vi "AguaClara Design Tool.vi"() -> ()   [LabVIEW 2015, in "AguaClara Library.lvlib"]
uses:
  AguaClara Library.lvlib
  Project commands.ctl
  language cmd.ctl
  Language.ctl
  User status cmd.ctl
  ADT Commands.ctl
  <vilib>/Utility/config.llb/NI_LVConfig.lvlib
  <vilib>/Utility/config.llb/Write Key (I32).vi
  <vilib>/Utility/config.llb/Read Key (I32).vi
  GUI controls commands.ctl
  <vilib>/Platform/browser.llb/Open URL in Default Browser (string).vi
  Project inputs.ctl
  toolbar icons/help.ctl
  User Information.ctl
  Basic Inputs.ctl
  Country Ring.ctl
panel:
  out "Quit now":bool caption="Terminar"
  in  "MSG Server unavailable":string caption="Disculpe. El servidor de AguaClara no está disponible."
  in  "MSG Design sent postcity":string caption="se ha enviado al servidor de AguaClara para el diseño. Los archivos serán enviados a su correo electrónico."
  in  "MSG Design sent precity":string caption="Su solicitude para la ciudad de"
  out "Design Inputs Label":string caption="Datos basicos"
  out "Project Info label":string caption="Información del proyecto"
  in  "Design Plant":bool caption="Mandar la solicitud"
  in  "Logon":bool caption="Entrar al sistema"
  in  "Log off":bool caption="Cierre la sesión"
  in  "Quit":bool caption="Terminar"
  in  "Project commands":T1 caption="Mandados del proyecto"
  in  "Project List":i32(listbox)=-1 caption="Lista de proyectos"
  in  "Help Button":T2 caption="Botón para ayuda"
  in  "Tab Control":enum32{" ", "  ", "Advanced Controls"}(tab)=enum."Advanced Controls" caption="Control de etiqueta"
  out "Project Info":T3 caption="Información del proyecto"
  out "Project date":timestamp[](array[timestamp]) caption="Fecha (dd/mm/aa)" format="%<%.3X\n%d/%m/%Y>T"
  out "User Information":T4 caption="Información del usuario" {"Country" items=["Afghanistan", "Aland Islands", "Albania", "Algeria", "American Samoa", "Andorra", "Angola", "Anguilla", "Antarctica", "Antigua And Barbuda", "Argentina", "Armenia", "Aruba", "Australia", "Austria", "Azerbaijan", "Bahamas", "Bahrain", "Bangladesh", "Barbados", "Belarus", "Belgium", "Belize", "Benin", "Bermuda", "Bhutan", "Bolivia", "Bosnia And Herzegovina", "Botswana", "Bouvet Island", "Brazil", "British Indian Ocean Territory", "Brunei Darussalam", "Bulgaria", "Burkina Faso", "Burundi", "Cambodia", "Cameroon", "Canada", "Cape Verde", "Cayman Islands", "Central African Republic", "Chad", "Chile", "China", "Christmas Island", "Cocos (Keeling) Islands", "Colombia", "Comoros", "Congo", "Congo, The Democratic Republic Of The", "Cook Islands", "Costa Rica", "Cote D'Ivoire", "Croatia", "Cuba", "Cyprus", "Czech Republic", "Denmark", "Djibouti", "Dominica", "Dominican Republic", "Ecuador", "Egypt", "El Salvador", "Equatorial Guinea", "Eritrea", "Estonia", "Ethiopia", "Falkland Islands (Malvinas)", "Faroe Islands", "Fiji", "Finland", "France", "French Guiana", "French Polynesia", "French Southern Territories", "Gabon", "Gambia", "Georgia", "Germany", "Ghana", "Gibraltar", "Greece", "Greenland", "Grenada", "Guadeloupe", "Guam", "Guatemala", "Guernsey", "Guinea", "Guinea-Bissau", "Guyana", "Haiti", "Heard Island And Mcdonald Islands", "Holy See (Vatican City State)", "Honduras", "Hong Kong", "Hungary", "Iceland", "India", "Indonesia", "Iran, Islamic Republic Of", "Iraq", "Ireland", "Isle Of Man", "Israel", "Italy", "Jamaica", "Japan", "Jersey", "Jordan", "Kazakhstan", "Kenya", "Kiribati", "Korea, Democratic People'S Republic Of", "Korea, Republic Of", "Kuwait", "Kyrgyzstan", "Lao People'S Democratic Republic", "Latvia", "Lebanon", "Lesotho", "Liberia", "Libyan Arab Jamahiriya", "Liechtenstein", "Lithuania", "Luxembourg", "Macao", "Macedonia, The Former Yugoslav Republic Of", "Madagascar", "Malawi", "Malaysia", "Maldives", "Mali", "Malta", "Marshall Islands", "Martinique", "Mauritania", "Mauritius", "Mayotte", "Mexico", "Micronesia, Federated States Of", "Moldova, Republic Of", "Monaco", "Mongolia", "Montserrat", "Morocco", "Mozambique", "Myanmar", "Namibia", "Nauru", "Nepal", "Netherlands", "Netherlands Antilles", "New Caledonia", "New Zealand", "Nicaragua", "Niger", "Nigeria", "Niue", "Norfolk Island", "Northern Mariana Islands", "Norway", "Oman", "Pakistan", "Palau", "Palestinian Territory, Occupied", "Panama", "Papua New Guinea", "Paraguay", "Peru", "Philippines", "Pitcairn", "Poland", "Portugal", "Puerto Rico", "Qatar", "Reunion", "Romania", "Russian Federation", "Rwanda", "Saint Helena", "Saint Kitts And Nevis", "Saint Lucia", "Saint Pierre And Miquelon", "Saint Vincent And The Grenadines", "Samoa", "San Marino", "Sao Tome And Principe", "Saudi Arabia", "Senegal", "Serbia And Montenegro", "Seychelles", "Sierra Leone", "Singapore", "Slovakia", "Slovenia", "Solomon Islands", "Somalia", "South Africa", "South Georgia And The South Sandwich Islands", "Spain", "Sri Lanka", "Sudan", "Suriname", "Svalbard And Jan Mayen", "Swaziland", "Sweden", "Switzerland", "Syrian Arab Republic", "Taiwan, Province Of China", "Tajikistan", "Tanzania, United Republic Of", "Thailand", "Timor-Leste", "Togo", "Tokelau", "Tonga", "Trinidad And Tobago", "Tunisia", "Turkey", "Turkmenistan", "Turks And Caicos Islands", "Tuvalu", "Uganda", "Ukraine", "United Arab Emirates", "United Kingdom", "United States", "United States Minor Outlying Islands", "Uruguay", "Uzbekistan", "Vanuatu", "Venezuela", "Viet Nam", "Virgin Islands, British", "Virgin Islands, U.S.", "Wallis And Futuna", "Western Sahara", "Yemen", "Zambia", "Zimbabwe", "(Not Specified)"]}
  out "Design Inputs":T6={"Q.Plant"=0.05, "C.CoagDoseMax"=0.01, "C.CoagStock"=0.01, "Ti.CoagStock"=0.0015, "EN.DrillSeries"=enum."English", "EN.TubeSeries"=enum."English", "N.SedTanks"=10.0, "N.SedBaysEst"=120.0, "W.SedPlate"=0.005, "L.SedPlateSheet"=0.0, "T.SedPlate"=388800000.0, "T.PlantWall"=0.03, "H.FlocOption"=0.01, "T.FlocBaffleRigidH"=0.03, "T.ConcreteMin"=0.3, "T.SedWeir"=0.3, "T.FlocBaffleRigidV"=108000.0} caption="Datos basicos" {"T.FlocBaffleRigidV" min=0.0 max=0.2 step=0.001 format="%#.1f"; "T.SedWeir" min=0.001 max=0.2 step=0.001 format="%#.1f"; "T.SedPlate" min=0.001 max=0.05 step=0.001 format="%#.1f"; "T.FlocBaffleRigidH" min=0.0 max=0.2 step=0.001 format="%#.1f"; "T.ConcreteMin" min=0.005 max=0.2 step=0.001 format="%#.1f"; "L.SedPlateSheet" min=0.3 max=8.0 step=0.01 format="%#.1f"; "N.SedBaysEst" min=1.0 max=20.0 step=1.0 format="%#.0f"; "N.SedTanks" min=1.0 max=20.0 step=1.0 format="%#.0f"; "Ti.CoagStock" min=43200.0 max=360000.0 step=3600.0 format="%#.1f"; "H.FlocOption" min=0.5 max=4.0 step=0.01 format="%#.2f"; "C.CoagStock" min=50.0 max=500.0 step=1.0 format="%#.0f"; "C.CoagDoseMax" min=0.03 max=0.2 step=0.005 format="%#.0f"; "Q.Plant" min=0.001 max=0.2 step=0.0001 format="%#.1f"; "T.PlantWall" min=0.05 max=0.5 step=0.001 format="%#.1f"; "W.SedPlate" min=0.5 max=3.0 step=0.001 format="%#.1f"}
  in  "Restart ADT":bool
  in  "Choose Server":bool
  in  "ADT version":i32 min=0 step=1
  in  "CheckOut ADT":bool
  in  "Translate":bool caption="Traducir"
  out "error out":errorcluster
  in  "Language":T7 caption="Idioma"
  out "design server":string="aguaclaraserver.cee.cornell.edu"
  out "File List":i32(listbox) caption="Lista de archivos"
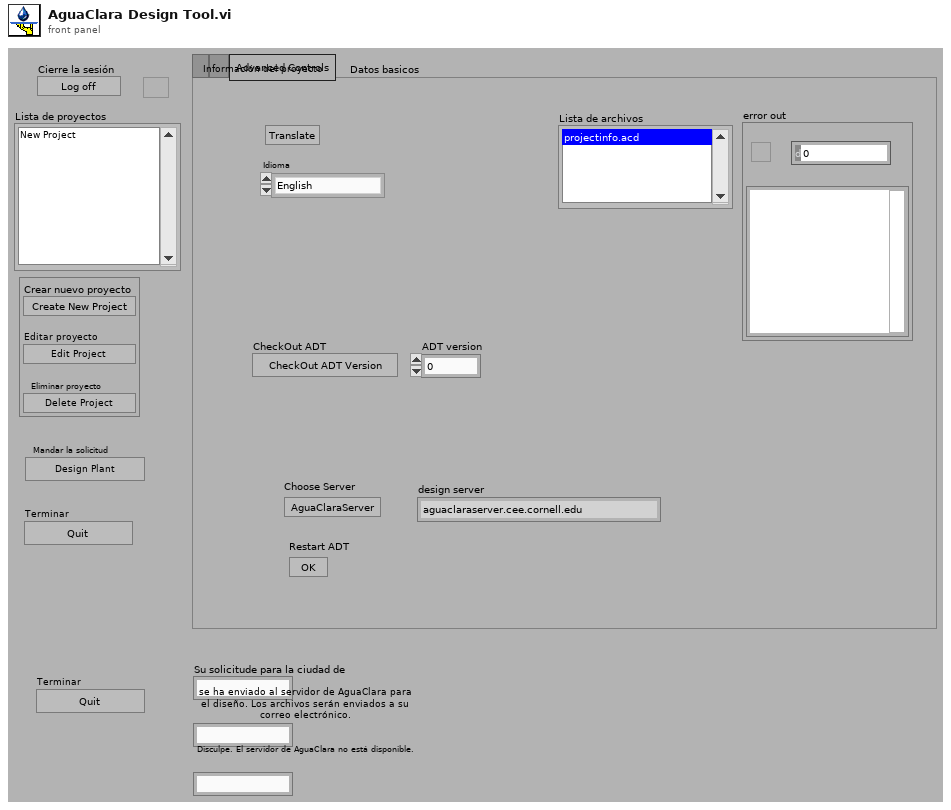
[diagram p1: front panel]
types:
  T1 = cluster{"Create New Project":bool, "Edit Project":bool, "Delete Project":bool}
  T2 = typedef "help.ctl" = bool
  T3 = typedef "AguaClara Library.lvlib/Project inputs.ctl" = cluster{"Project Name":string, "City":string, "State":string, "Notes":string}
  T4 = typedef "AguaClara Library.lvlib/User Information.ctl" = cluster{"First Name":string, "Last Name":string, "Email Address":string, "Organization":string, "Language":enum16{"English", "Español", "French"}, "Country":T5}
  T5 = typedef "Country Ring.ctl" = u16
  T6 = typedef "AguaClara Library.lvlib/Basic Inputs.ctl" = cluster{"Q.Plant":dbl[unit], "C.CoagDoseMax":dbl[unit], "C.CoagStock":dbl[unit], "Ti.CoagStock":dbl[unit], "EN.DrillSeries":enum16{"English", "Metric"}, "EN.TubeSeries":enum16{"English", "Metric"}, "N.SedTanks":dbl, "N.SedBaysEst":dbl, "W.SedPlate":dbl[unit], "L.SedPlateSheet":dbl[unit], "T.SedPlate":dbl[unit], "T.PlantWall":dbl[unit], "H.FlocOption":dbl[unit], "T.FlocBaffleRigidH":dbl[unit], "T.ConcreteMin":dbl[unit], "T.SedWeir":dbl[unit], "T.FlocBaffleRigidV":dbl[unit]}
  T7 = typedef "AguaClara Library.lvlib/Language.ctl" = enum16{"English", "Español", "French"}
  T8 = typedef "GUI controls commands.ctl" = enum16{"Load controls", "Set controls"}
  T9 = typedef "AguaClara Library.lvlib/User status cmd.ctl" = enum16{"Load File Path", "Create account", "Update user", "Email password", "Load inputs", "Check status"}
  T10 = typedef "AguaClara Library.lvlib/language cmd.ctl" = enum16{"load inputs", "choose language", "translate", "load storage variable from file"}
  T11 = typedef "AguaClara Library.lvlib/Project commands.ctl" = enum16{"Load base file", "Load User", "Read paths", "Open Project", "New project", "Edit project", "Delete project", "Mail project", "save design", "open design"}
  T12 = typedef "ADT Commands.ctl" = enum16{"Design Plant", "CheckOut MathCAD Files", "Restart"}
  T13 = typedef "NI_LVConfig.lvlib/Config Data RefNum.ctl" = refnum<k1>
  T14 = typedef "packed var.ctl" = variant
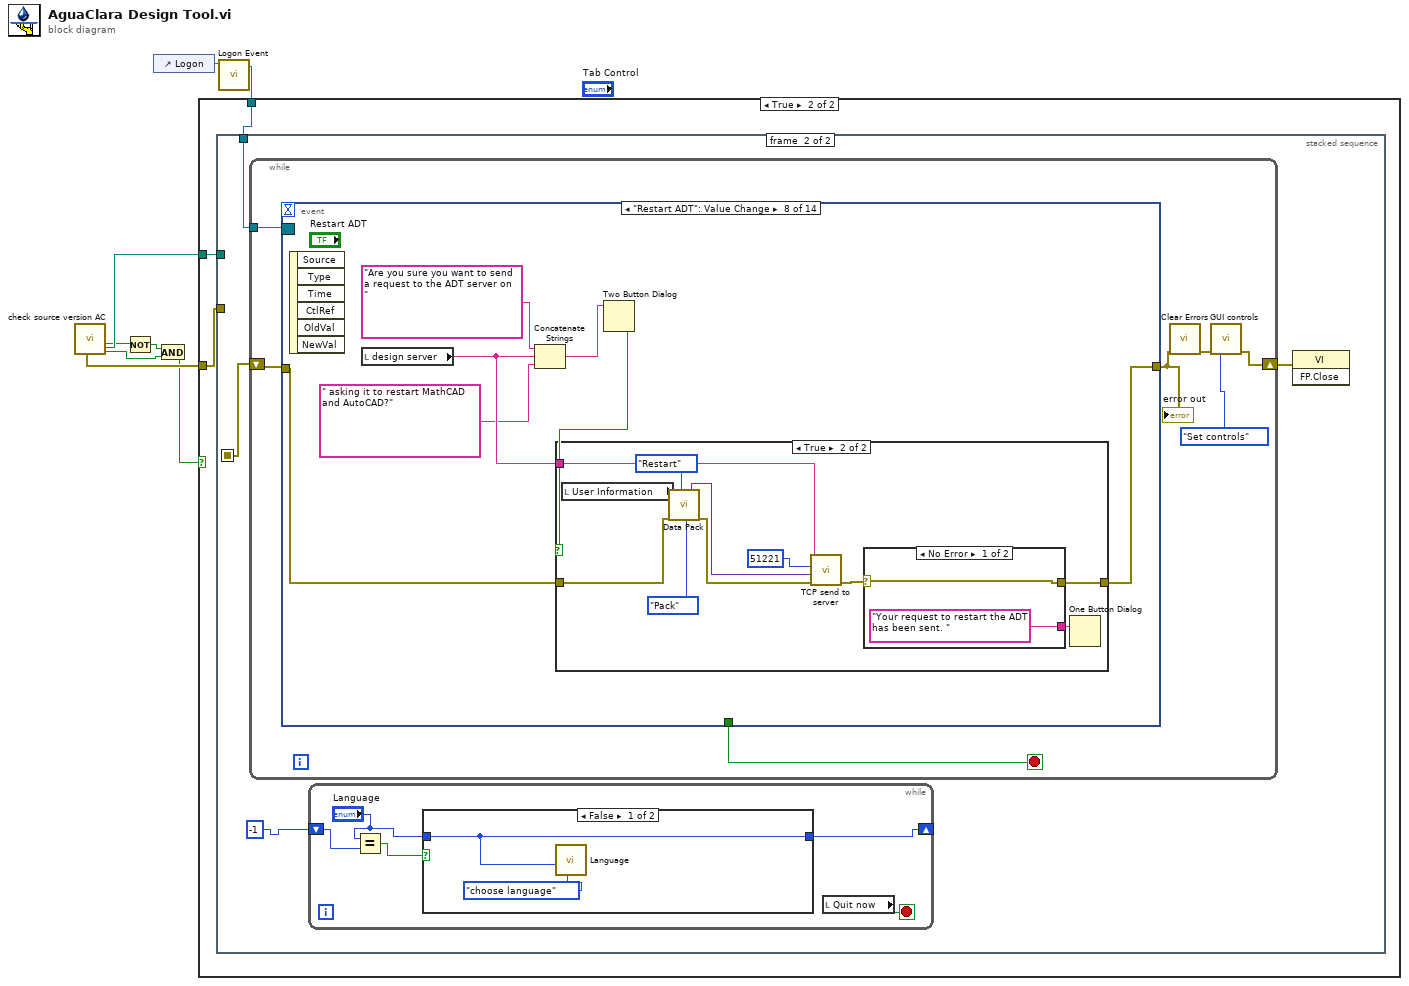
[diagram p0: block diagram]
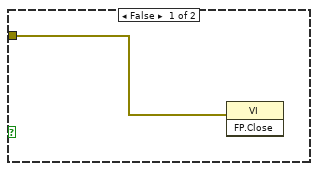
[diagram p2: hidden frame]
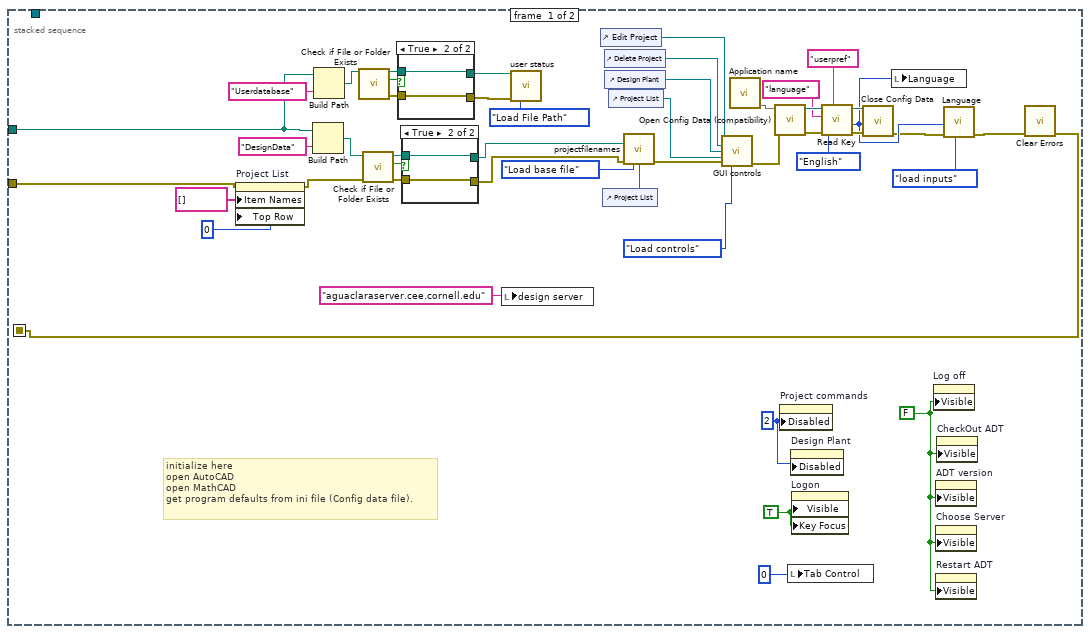
[diagram p3: hidden frame]
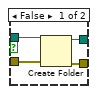
[diagram p4: hidden frame]
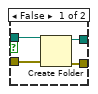
[diagram p5: hidden frame]
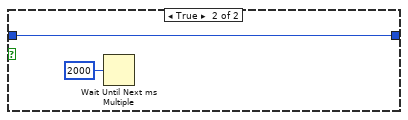
[diagram p6: hidden frame]
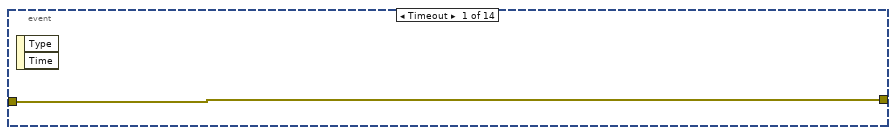
[diagram p7: hidden frame]
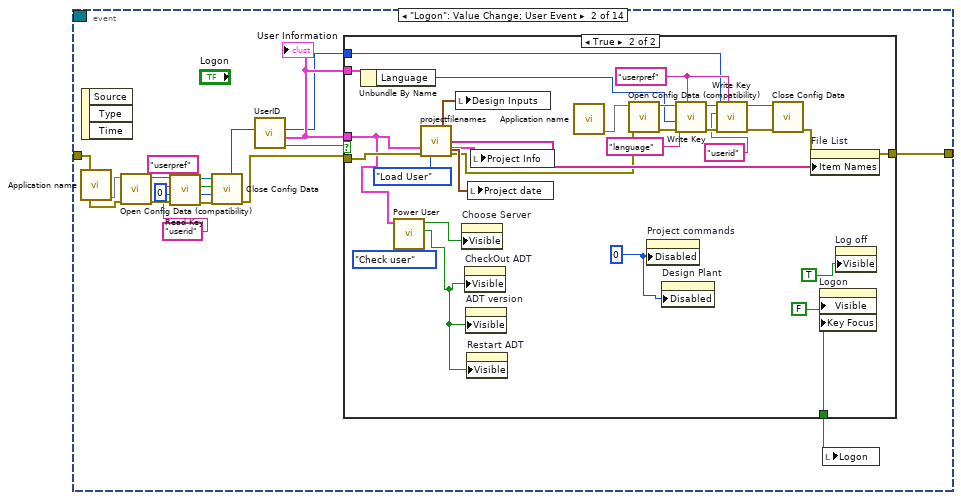
[diagram p8: hidden frame]
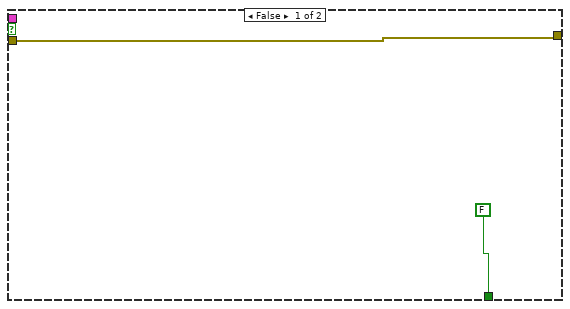
[diagram p9: hidden frame]
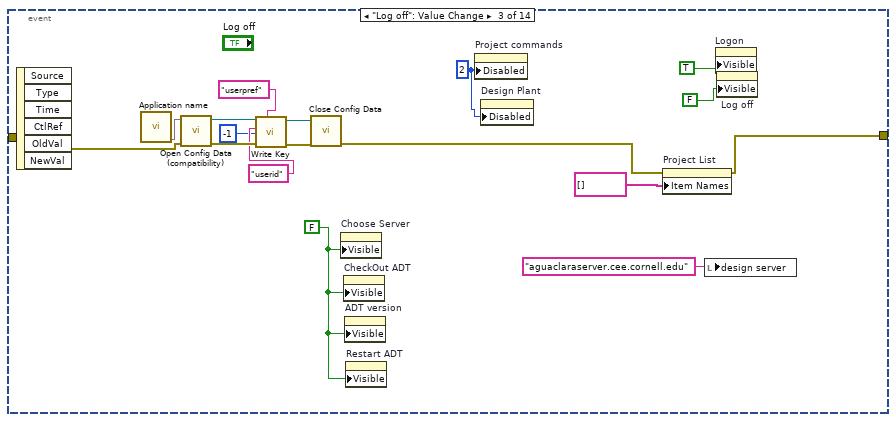
[diagram p10: hidden frame]
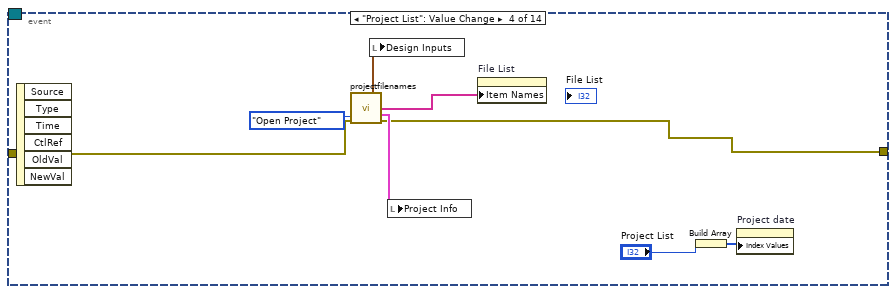
[diagram p11: hidden frame]
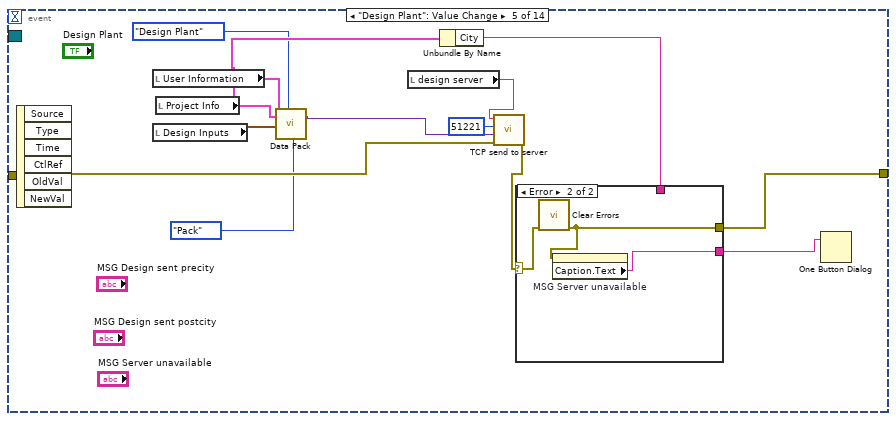
[diagram p12: hidden frame]
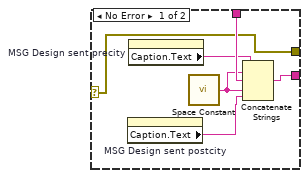
[diagram p13: hidden frame]
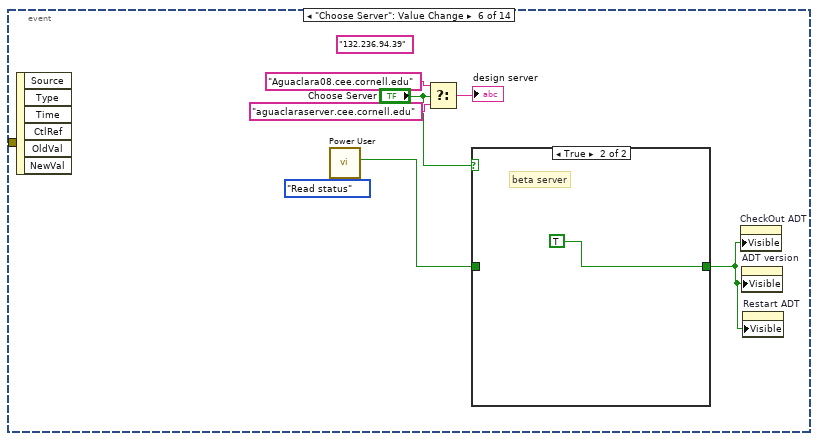
[diagram p14: hidden frame]
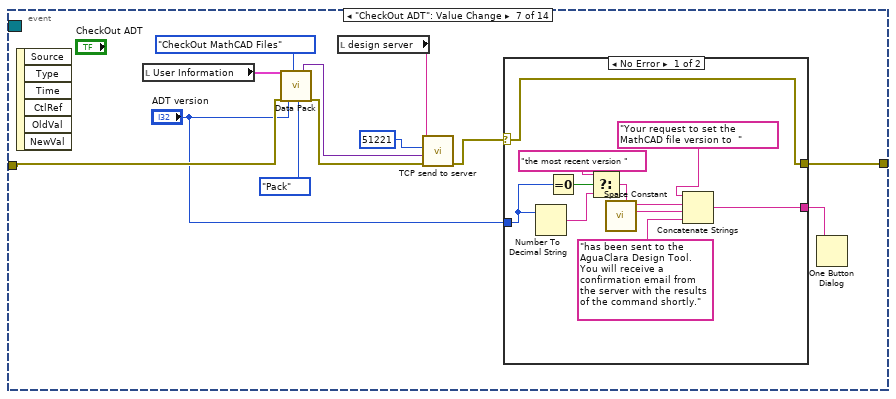
[diagram p16: hidden frame]
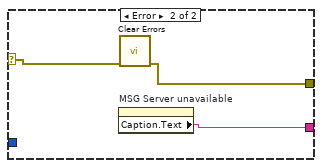
[diagram p17: hidden frame]
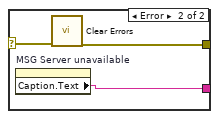
[diagram p19: hidden frame]
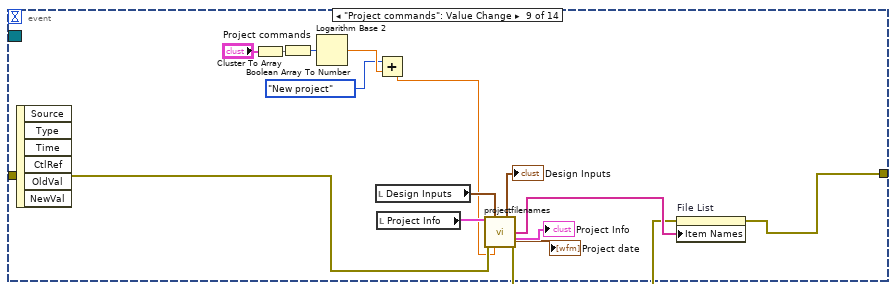
[diagram p20: hidden frame]
diagram:
  n1 = call "check source version AC.vi"() -> ("continue running?"=w2:bool, "Newer version available"=w4:bool, "Application folder"=w8:path, "error out"=w7:errorcluster)  [unwired: 3 in, 5 out]
  n2 = Not(x=w4) -> (.not. x?=w3:bool)
  n3 = control-ref of="Logon"() -> (w6:refnum<vi>)
  n4 = And(x=w3, y=w2) -> (x .and. y?=w1:bool)
  n5 = call "Logon Event.vi"("reference"=w6) -> ("Event Registration Refnum"=w5:refnum<event-registration>)  [unwired: 10 in]
  n6 = case shown="True" w1 {
    tunnel: w8 -> [_ w12]
    tunnel: w7 -> [w9 w11]
    tunnel: w5 -> [_ w10]
    frame False {
      n7 = invoke class="VI" method="FP.Close"(error in=w9) -> ()  [unwired: 2 in, 3 out]
    }
    frame True {
      n8 = stacked-sequence {
        seq-local: [w33 _] -> [_ w75]
        tunnel: w12 -> [w51 _]
        tunnel: w11 -> [w32 _]
        tunnel: w10 -> [_ w74]
        frame #0 {
          w13 = FALSE ("Visible")
          w56 = TRUE ("Visible")
          w48 = u8 2 ("Disabled")
          # "initialize here\nopen AutoCAD\nopen MathCAD\nget program defaults from ini file (Config data file)."
          n9 = property on="Project List" class="LstBox (strict)"(error in=w32, "Item Names"=string[] [], "Top Row"=0) -> (error out=w35:errorcluster)  [unwired: 1 in, 1 out]
          n10 = Build Path(base path=w51, name or relative path="DesignData") -> (appended path=w38:path)
          n11 = Build Path(base path=w51, name or relative path="Userdatabase") -> (appended path=w42:path)
          n12 = call <vilib>:"Check if File or Folder Exists.vi"("path"=w42) -> ("error out"=w47:errorcluster, "file or folder exists?"=w45:bool, "dup path"=w46:path)  [unwired: 8 in]
          n13 = call <vilib>:"Check if File or Folder Exists.vi"("error in (no error)"=w35, "path"=w38) -> ("error out"=w41:errorcluster, "file or folder exists?"=w39:bool, "dup path"=w40:path)  [unwired: 7 in]
          n14 = case shown="True" w45 {
            tunnel: w47 -> [w69 w70]
            tunnel: w46 -> [w68 w71]
            tunnel: [w67 w71] -> w44
            tunnel: [w66 w70] -> w43
            frame False {
              n15 = Create Folder(path (use dialog)=w68, error in=w69) -> (created path=w67:path, error out=w66:errorcluster)  [unwired: 1 in, 1 out]
            }
            frame True {
            }
          }
          n16 = case shown="True" w39 {
            tunnel: w41 -> [w63 w64]
            tunnel: w40 -> [w62 w65]
            tunnel: [w61 w65] -> w37
            tunnel: [w60 w64] -> w36
            frame False {
              n17 = Create Folder(path (use dialog)=w62, error in=w63) -> (created path=w61:path, error out=w60:errorcluster)  [unwired: 1 in, 1 out]
            }
            frame True {
            }
          }
          n18 = local write "design server"("aguaclaraserver.cee.cornell.edu" ("Machine")) -> ()
          n19 = call "user status.vi"("Userdatabase"=w44, "error in (no error)"=w43, "User status cmd"=User_status_cmd."Load File Path") -> ()  [unwired: 8 in, 5 out]
          n20 = control-ref of="Edit Project"() -> (w20:refnum<vi>)
          n21 = control-ref of="Project List"() -> (w57:refnum<vi>)
          n22 = control-ref of="Delete Project"() -> (w17:refnum<vi>)
          n23 = control-ref of="Design Plant"() -> (w16:refnum<vi>)
          n24 = control-ref of="Project List"() -> (w15:refnum<vi>)
          n25 = call "projectfilenames.vi"("Base File Path"=w37, "error in (no error)"=w36, "Project command"=Project_commands."Load base file", "LstBox Refnum"=w57) -> ("error out"=w22:errorcluster)  [unwired: 6 in, 5 out]
          n26 = call "GUI controls.vi"("Edit"=w20, "Delete"=w17, "Design"=w16, "Project List"=w15, "error in (no error)"=w22, "GUI controls commands"=GUI_controls_commands."Load controls") -> ("error out"=w19:errorcluster)  [unwired: 9 in]
          n27 = call "Application name.vi"() -> (0:w31)  [unwired: 4 in, 3 out]
          n28 = call <vilib>:"Open Config Data (compatibility).vi"("error in (no error)"=w19, "configuration file path"=w31) -> ("error out"=w30:errorcluster, "refnum"=w29:T13)  [unwired: 7 in, 1 out]
          n29 = property on="Project commands" class="Clust"("Disabled"=w48) -> ()  [unwired: 2 in, 2 out]
          n30 = local write "Tab Control"(u8 0 ("Disabled")) -> ()
          n31 = property on="Design Plant" class="Bool"("Disabled"=w48) -> ()  [unwired: 2 in, 2 out]
          n32 = property on="Logon" class="Bool (strict)"("Visible"=w56, "Key Focus"=w56) -> ()  [unwired: 2 in, 2 out]
          n33 = call-poly <vilib>:"Read Key.vi"("section"="userpref", "error in (no error)"=w30, "default value"=Language."English" ("Language"), "key"="language", "refnum"=w29) -> ("error out"=w28:errorcluster, "value"=w23:i32, "refnum out"=w27:T13)  [unwired: 3 in, 1 out]
          n34 = call <vilib>:"Close Config Data.vi"("error in (no error)"=w28, "refnum"=w27) -> ("error out"=w18:errorcluster)  [unwired: 8 in, 1 out]
          n35 = local write "Language"(w23) -> ()
          n36 = property on="Log off" class="Bool"("Visible"=w13) -> ()  [unwired: 2 in, 2 out]
          n37 = property on="ADT version" class="DigNum (strict)"("Visible"=w13) -> ()  [unwired: 2 in, 2 out]
          n38 = property on="Choose Server" class="Bool (strict)"("Visible"=w13) -> ()  [unwired: 2 in, 2 out]
          n39 = property on="Restart ADT" class="Bool"("Visible"=w13) -> ()  [unwired: 2 in, 2 out]
          n40 = property on="CheckOut ADT" class="Bool"("Visible"=w13) -> ()  [unwired: 2 in, 2 out]
          n41 = call "Language.vi"("language cmd"=language_cmd."load inputs", "error in (no error)"=w18, "Language"=w23) -> ("error out"=w54:errorcluster)  [unwired: 7 in, 1 out]
          n42 = call <vilib>:"Clear Errors.vi"("error in (no error)"=w54) -> ("error out"=w33:errorcluster)  [unwired: 5 in, 1 out]
        }
        frame #1 {
          n43 = while {
            shift-right: [w86] -> w73
            shift-left: w75 -> [w90]
            tunnel: w74 -> [w88]
            stop <- w91 stop-if-true
            n44 = event shown="[7] \"Restart ADT\": Value Change" {
              selector: w88 -> [_ _ _ _ _ _ _ _ _ _ _ _ _ _]
              dyn-events: _ -> [_ _ _ _ _ _ _ _ _ _ _ _ _ _]
              timeout: _ -> [_ _ _ _ _ _ _ _ _ _ _ _ _ _]
              tunnel: [_ _ _ _ _ _ _ _ _ _ _ _ _ w269] -> w91
              tunnel: [w92 w108 w143 w158 w173 _ w198 w227 w249 _ _ w263 w266 _] -> w89
              tunnel: w90 -> [w92 w94 w145 w159 w177 _ w205 w228 w251 _ _ w264 w267 _]
              event Timeout {
                n45 = event-data() -> ()  [unwired: 1 in, 2 out]
              }
              event "Logon": Value Change; User Event {
                n46 = call "Application name.vi"() -> (0:w104)  [unwired: 4 in, 3 out]
                n47 = event-data() -> ()  [unwired: 1 in, 3 out]
                n48 = call <vilib>:"Open Config Data (compatibility).vi"("error in (no error)"=w94, "configuration file path"=w104) -> ("error out"=w103:errorcluster, "refnum"=w102:T13)  [unwired: 7 in, 1 out]
                n49 = call-poly <vilib>:"Read Key.vi"("section"="userpref", "error in (no error)"=w103, "default value"=0 ("User Index"), "key"="userid", "refnum"=w102) -> ("error out"=w97:errorcluster, "value"=w98:i32, "found?"=w96:bool, "refnum out"=w95:T13)  [unwired: 3 in]
                n50 = call <vilib>:"Close Config Data.vi"("error in (no error)"=w97, "write file if changed (T)"=w96, "refnum"=w95) -> ("error out"=w93:errorcluster)  [unwired: 7 in, 1 out]
                n51 = call "UserID.vi"("User Index in"=w98) -> ("valid user"=w109:bool, "User Information out"=w106:T4, "User Index out"=w105:i32)  [unwired: 8 in]
                "User Information" <- w106
                n52 = case shown="True" w109 {
                  tunnel: w106 -> [_ w131]
                  tunnel: [w111 w132] -> w108
                  tunnel: w93 -> [w111 w134]
                  tunnel: [FALSE ("Visible") w130] -> w107
                  tunnel: w106 -> [_ w129]
                  tunnel: w105 -> [_ w116]
                  frame False {
                  }
                  frame True {
                    w130 = FALSE ("Visible")
                    w133 = u8 0 ("Disabled")
                    w118 = "userpref" ("section")
                    n53 = Unbundle By Name(w129) -> ("Language"=w124:enum16{"English", "Español", "French"})
                    n54 = call "Power User.vi"("PowerUser"=enum16{"Check user", "Read status"}."Check user", "User Information"=w131) -> ("Power User"=w121:bool, "Cornell User"=w123:bool)  [unwired: 8 in]
                    n55 = call "projectfilenames.vi"("User Information"=w131, "error in (no error)"=w134, "Project command"=Project_commands."Load User") -> ("Design Inputs out"=w136:T6, "File List"=w135:string[], "Project Info out"=w137:T3, "Project dates"=w139:timestamp[], "error out"=w113:errorcluster)  [unwired: 7 in, 1 out]
                    n56 = local write "Design Inputs"(w136) -> ()
                    n57 = property on="Choose Server" class="Bool (strict)"("Visible"=w123) -> ()  [unwired: 2 in, 2 out]
                    n58 = property on="CheckOut ADT" class="Bool"("Visible"=w121) -> ()  [unwired: 2 in, 2 out]
                    n59 = property on="ADT version" class="DigNum (strict)"("Visible"=w121) -> ()  [unwired: 2 in, 2 out]
                    n60 = property on="Restart ADT" class="Bool"("Visible"=w121) -> ()  [unwired: 2 in, 2 out]
                    n61 = local write "Project date"(w139) -> ()
                    n62 = local write "Project Info"(w137) -> ()
                    n63 = call "Application name.vi"() -> (0:w128)  [unwired: 4 in, 3 out]
                    n64 = call <vilib>:"Open Config Data (compatibility).vi"("error in (no error)"=w113, "configuration file path"=w128) -> ("error out"=w127:errorcluster, "refnum"=w126:T13)  [unwired: 7 in, 1 out]
                    n65 = property on="Project commands" class="Clust"("Disabled"=w133) -> ()  [unwired: 2 in, 2 out]
                    n66 = property on="Design Plant" class="Bool"("Disabled"=w133) -> ()  [unwired: 2 in, 2 out]
                    n67 = call-poly <vilib>:"Write Key.vi"("section"=w118, "error in (no error)"=w127, "value"=w124, "key"="language", "refnum"=w126) -> ("error out"=w120:errorcluster, "refnum out"=w119:T13)  [unwired: 4 in, 1 out]
                    n68 = call-poly <vilib>:"Write Key.vi"("section"=w118, "error in (no error)"=w120, "value"=w116, "key"="userid", "refnum"=w119) -> ("error out"=w114:errorcluster, "refnum out"=w115:T13)  [unwired: 4 in, 1 out]
                    n69 = call <vilib>:"Close Config Data.vi"("error in (no error)"=w114, "refnum"=w115) -> ("error out"=w112:errorcluster)  [unwired: 8 in, 1 out]
                    n70 = property on="File List" class="LstBox (strict)"(error in=w112, "Item Names"=w135) -> (error out=w132:errorcluster)  [unwired: 1 in, 1 out]
                    n71 = property on="Logon" class="Bool (strict)"("Visible"=w130, "Key Focus"=w130) -> ()  [unwired: 2 in, 2 out]
                    n72 = property on="Log off" class="Bool"("Visible"=TRUE) -> ()  [unwired: 2 in, 2 out]
                  }
                }
                n73 = local write "Logon"(w107) -> ()
              }
              event "Log off": Value Change {
                w154 = u8 2 ("Disabled")
                w153 = FALSE ("Visible")
                n74 = event-data() -> ()  [unwired: 1 in, 6 out]
                n75 = call "Application name.vi"() -> (0:w151)  [unwired: 4 in, 3 out]
                n76 = call <vilib>:"Open Config Data (compatibility).vi"("error in (no error)"=w145, "configuration file path"=w151) -> ("error out"=w150:errorcluster, "refnum"=w149:T13)  [unwired: 7 in, 1 out]
                n77 = call-poly <vilib>:"Write Key.vi"("section"="userpref", "error in (no error)"=w150, "value"=-1 ("User Index"), "key"="userid", "refnum"=w149) -> ("error out"=w147:errorcluster, "refnum out"=w146:T13)  [unwired: 4 in, 1 out]
                n78 = call <vilib>:"Close Config Data.vi"("error in (no error)"=w147, "refnum"=w146) -> ("error out"=w144:errorcluster)  [unwired: 8 in, 1 out]
                n79 = property on="Choose Server" class="Bool (strict)"("Visible"=w153) -> ()  [unwired: 2 in, 2 out]
                n80 = property on="CheckOut ADT" class="Bool"("Visible"=w153) -> ()  [unwired: 2 in, 2 out]
                n81 = property on="ADT version" class="DigNum (strict)"("Visible"=w153) -> ()  [unwired: 2 in, 2 out]
                n82 = property on="Restart ADT" class="Bool"("Visible"=w153) -> ()  [unwired: 2 in, 2 out]
                n83 = property on="Project commands" class="Clust"("Disabled"=w154) -> ()  [unwired: 2 in, 2 out]
                n84 = property on="Design Plant" class="Bool"("Disabled"=w154) -> ()  [unwired: 2 in, 2 out]
                n85 = property on="Project List" class="LstBox (strict)"(error in=w144, "Item Names"=string[] []) -> (error out=w143:errorcluster)  [unwired: 1 in, 1 out]
                n86 = local write "design server"("aguaclaraserver.cee.cornell.edu" ("Machine")) -> ()
                n87 = property on="Logon" class="Bool (strict)"("Visible"=TRUE) -> ()  [unwired: 2 in, 2 out]
                n88 = property on="Log off" class="Bool"("Visible"=FALSE) -> ()  [unwired: 2 in, 2 out]
              }
              event "Project List": Value Change {
                n89 = event-data() -> ()  [unwired: 1 in, 6 out]
                n90 = call "projectfilenames.vi"("error in (no error)"=w159, "Project command"=Project_commands."Open Project") -> ("Design Inputs out"=w164:T6, "File List"=w160:string[], "Project Info out"=w163:T3, "error out"=w158:errorcluster)  [unwired: 8 in, 2 out]
                n91 = local write "Design Inputs"(w164) -> ()
                n92 = local write "Project Info"(w163) -> ()
                n93 = property on="File List" class="LstBox (strict)"("Item Names"=w160) -> ()  [unwired: 2 in, 2 out]
                n94 = Build Array("Project List") -> (w161:i32[])
                n95 = property on="Project date" class="Arr (strict)"("Index Values"=w161) -> ()  [unwired: 2 in, 2 out]
              }
              event "Design Plant": Value Change {
                n96 = event-data() -> ()  [unwired: 1 in, 6 out]
                n97 = local read "User Information"() -> (w169:T4)
                n98 = local read "Design Inputs"() -> (w171:T6)
                n99 = local read "Project Info"() -> (w170:T3)
                n100 = call "Data Pack.vi"("User Information"=w169, "Project Info"=w170, "Design Inputs"=w171, "ADT Commands"=ADT_Commands."Design Plant", "Data transform"=enum16{"Pack", "UnPack"}."Pack") -> ("Packed Out"=w168:T14)  [unwired: 7 in, 7 out]
                n101 = local read "design server"() -> (w166:string)
                n102 = Unbundle By Name(w170) -> ("City"=w178:string)
                n103 = call "TCP send to server.vi"("error in (no error)"=w177, "Packed In"=w168, "Port"=u16 51221, "Machine"=w166) -> ("error out"=w174:errorcluster)  [unwired: 6 in, 1 out]
                n104 = case shown="Error" w174 {
                  selector: w174 -> [w179 w186]
                  tunnel: w178 -> [w184 _]
                  tunnel: [w180 w187] -> w175
                  tunnel: [w179 w185] -> w173
                  frame No Error {
                    n105 = property on="MSG Design sent postcity" class="Str"() -> ("Caption.Text"=w182:string)  [unwired: 2 in, 2 out]
                    n106 = property on="MSG Design sent precity" class="Str"() -> ("Caption.Text"=w181:string)  [unwired: 2 in, 2 out]
                    n107 = call <vilib>:"Space Constant.vi"() -> ("String"=w183:string)
                    n108 = Concatenate Strings(w181, w183, w184, w183, w182) -> (w180:string)
                  }
                  frame Error {
                    n109 = call <vilib>:"Clear Errors.vi"("error in (no error)"=w186) -> ("error out"=w185:errorcluster)  [unwired: 5 in, 1 out]
                    n110 = property on="MSG Server unavailable" class="Str"(error in=w185) -> ("Caption.Text"=w187:string)  [unwired: 1 in, 2 out]
                  }
                }
                n111 = One Button Dialog(message=w175) -> ()  [unwired: 1 in, 1 out]
              }
              event "Choose Server": Value Change {
                (unwired) "132.236.94.39" ("Machine")
                n112 = event-data() -> ()  [unwired: 1 in, 6 out]
                n113 = call "Power User.vi"("PowerUser"=enum16{"Check user", "Read status"}."Read status") -> ("Power User"=w189:bool)  [unwired: 9 in, 1 out]
                n114 = Select(t="Aguaclara08.cee.cornell.edu" ("Machine"), s="Choose Server", f="aguaclaraserver.cee.cornell.edu" ("Machine")) -> (s? t:f=→"design server":string)
                n115 = case shown="True" "Choose Server" {
                  tunnel: [w195 TRUE ("Visible")] -> w190
                  tunnel: w189 -> [w195 _]
                  frame False {
                    # "official server"
                  }
                  frame True {
                    # "beta server"
                  }
                }
                n116 = property on="CheckOut ADT" class="Bool"("Visible"=w190) -> ()  [unwired: 2 in, 2 out]
                n117 = property on="ADT version" class="DigNum (strict)"("Visible"=w190) -> ()  [unwired: 2 in, 2 out]
                n118 = property on="Restart ADT" class="Bool"("Visible"=w190) -> ()  [unwired: 2 in, 2 out]
              }
              event "CheckOut ADT": Value Change {
                n119 = event-data() -> ()  [unwired: 1 in, 6 out]
                n120 = local read "User Information"() -> (w203:T4)
                n121 = call "Data Pack.vi"("User Information"=w203, "error in"=w205, "ADT version"="ADT version", "ADT Commands"=ADT_Commands."CheckOut MathCAD Files", "Data transform"=enum16{"Pack", "UnPack"}."Pack") -> ("Packed Out"=w206:T14, "error out"=w204:errorcluster)  [unwired: 7 in, 6 out]
                n122 = local read "design server"() -> (w197:string)
                n123 = call "TCP send to server.vi"("error in (no error)"=w204, "Packed In"=w206, "Port"=u16 51221, "Machine"=w197) -> ("error out"=w201:errorcluster)  [unwired: 6 in, 1 out]
                n124 = case shown="No Error" w201 {
                  selector: w201 -> [w209 w220]
                  tunnel: "ADT version" -> [w217 _]
                  tunnel: [w210 w221] -> w199
                  tunnel: [w209 w219] -> w198
                  frame No Error {
                    n125 = Number To Decimal String(number=w217) -> (decimal integer string=w215:string)  [unwired: 1 in]
                    n126 = Equal To 0?(x=w217) -> (x = 0?=w218:bool)
                    n127 = Select(t="the most recent version " ("message"), s=w218, f=w215) -> (s? t:f=w213:string)
                    n128 = call <vilib>:"Space Constant.vi"() -> ("String"=w212:string)
                    n129 = Concatenate Strings("Your request to set the MathCAD file version to  " ("message"), w213, w212, "has been sent to the AguaClara Design Tool. You will receive a confirmation email from the server with the results of the command shortly." ("string")) -> (w210:string)
                  }
                  frame Error {
                    n130 = property on="MSG Server unavailable" class="Str"() -> ("Caption.Text"=w221:string)  [unwired: 2 in, 2 out]
                    n131 = call <vilib>:"Clear Errors.vi"("error in (no error)"=w220) -> ("error out"=w219:errorcluster)  [unwired: 5 in, 1 out]
                  }
                }
                n132 = One Button Dialog(message=w199) -> ()  [unwired: 1 in, 1 out]
              }
              event "Restart ADT": Value Change {
                n133 = event-data() -> ()  [unwired: 1 in, 6 out]
                n134 = local read "design server"() -> (w224:string)
                n135 = Concatenate Strings("Are you sure you want to send a request to the ADT server on  " ("message"), w224, " asking it to restart MathCAD and AutoCAD?" ("message")) -> (w222:string)
                n136 = Two Button Dialog(message=w222) -> (T button?=w226:bool)  [unwired: 2 in]
                n137 = case shown="True" w226 {
                  tunnel: w228 -> [w229 w237]
                  tunnel: [w229 w231] -> w227
                  tunnel: w224 -> [_ w230]
                  frame False {
                  }
                  frame True {
                    n138 = local read "User Information"() -> (w235:T4)
                    n139 = call "Data Pack.vi"("User Information"=w235, "error in"=w237, "ADT Commands"=ADT_Commands."Restart", "Data transform"=enum16{"Pack", "UnPack"}."Pack") -> ("Packed Out"=w238:T14, "error out"=w236:errorcluster)  [unwired: 8 in, 6 out]
                    n140 = call "TCP send to server.vi"("error in (no error)"=w236, "Packed In"=w238, "Port"=u16 51221, "Machine"=w230) -> ("error out"=w233:errorcluster)  [unwired: 6 in, 1 out]
                    n141 = case shown="No Error" w233 {
                      selector: w233 -> [w242 w244]
                      tunnel: ["Your request to restart the ADT has been sent. " ("message") w245] -> w232
                      tunnel: [w242 w243] -> w231
                      frame No Error {
                      }
                      frame Error {
                        n142 = property on="MSG Server unavailable" class="Str"() -> ("Caption.Text"=w245:string)  [unwired: 2 in, 2 out]
                        n143 = call <vilib>:"Clear Errors.vi"("error in (no error)"=w244) -> ("error out"=w243:errorcluster)  [unwired: 5 in, 1 out]
                      }
                    }
                    n144 = One Button Dialog(message=w232) -> ()  [unwired: 1 in, 1 out]
                  }
                }
              }
              event "Project commands": Value Change {
                n145 = event-data() -> ()  [unwired: 1 in, 6 out]
                n146 = Cluster To Array(cluster="Project commands") -> (array=w260:bool[])
                n147 = Boolean Array To Number(Boolean array=w260) -> (number=w259:u32)
                n148 = Logarithm Base 2(1:w259) -> (0:w254:dbl)
                n149 = local read "Design Inputs"() -> (w256:T6)
                n150 = Add(x=Project_commands."New project" ("Project command"), y=w254) -> (x+y=w248:dbl)
                n151 = local read "Project Info"() -> (w257:T3)
                n152 = call "projectfilenames.vi"("Project Info"=w257, "Design Inputs"=w256, "error in (no error)"=w251, "Project command"=w248) -> ("Design Inputs out"=→"Design Inputs":T6, "File List"=w253:string[], "Project Info out"=→"Project Info":T3, "Project dates"=→"Project date":timestamp[], "error out"=w252:errorcluster)  [unwired: 6 in, 1 out]
                n153 = property on="File List" class="LstBox (strict)"(error in=w252, "Item Names"=w253) -> (error out=w249:errorcluster)  [unwired: 1 in, 1 out]
              }
              event "Project Info label": Mouse Up {
                n154 = event-data() -> ()  [unwired: 1 in, 8 out]
                n155 = local write "Tab Control"(0) -> ()
              }
              event "Design Inputs Label": Mouse Up {
                n156 = event-data() -> ()  [unwired: 1 in, 8 out]
                n157 = local write "Tab Control"(1) -> ()
              }
              event Value Change {
                # "This currently links to a wiki page where we are describing our programing strategy."
                n158 = event-data() -> ()  [unwired: 1 in, 6 out]
                n159 = call-poly <vilib>:"Open URL in Default Browser.vi"("error in (no error)"=w264, "URL"="https://confluence.cornell.edu/display/AGUACLARA/AguaClara+Design+Tool") -> ("error out"=w263:errorcluster)  [unwired: 4 in, 1 out]
              }
              event "Translate": Value Change {
                n160 = event-data() -> ()  [unwired: 1 in, 6 out]
                n161 = call "Language.vi"("language cmd"=language_cmd."translate", "error in (no error)"=w267) -> ("error out"=w266:errorcluster)  [unwired: 8 in, 1 out]
              }
              event "Quit": Value Change; Panel Close {
                w269 = TRUE ("Quit")
                n162 = event-data() -> ()  [unwired: 1 in, 3 out]
                "Quit now" <- w269
              }
            }
            "error out" <- w89
            n163 = call <vilib>:"Clear Errors.vi"("error in (no error)"=w89) -> ("error out"=w87:errorcluster)  [unwired: 5 in, 1 out]
            n164 = call "GUI controls.vi"("error in (no error)"=w87, "GUI controls commands"=GUI_controls_commands."Set controls") -> ("error out"=w86:errorcluster)  [unwired: 13 in]
          }
          n165 = while {
            shift-right: [w79] -> _
            shift-left: -1 -> [w77]
            stop <- w80 stop-if-true
            n166 = Equal?(x="Language", y=w77) -> (x = y?=w78:bool)
            n167 = case shown="False" w78 {
              tunnel: [w81 w84] -> w79
              tunnel: "Language" -> [w81 w84]
              frame False {
                n168 = call "Language.vi"("language cmd"=language_cmd."choose language", "Language"=w81) -> ()  [unwired: 8 in, 2 out]
              }
              frame True {
                n169 = Wait Until Next ms Multiple(millisecond multiple=u32 2000) -> ()  [unwired: 1 out]
              }
            }
            n170 = local read "Quit now"() -> (w80:bool)
          }
          n171 = invoke class="VI" method="FP.Close"(error in=w73) -> ()  [unwired: 2 in, 3 out]
        }
      }
    }
  }
